vi "Main.vi"(11 "Error in":errorcluster) -> (15 "Error out":errorcluster)   [LabVIEW 2020, in "Automated Teller Machine.lvlib"]
doc: "The ATM will simulate the actual working of a real time ATM machine which stores the customer credentials and the money available in a csv file."
uses:
  Automated Teller Machine.lvlib
  Type_def/Queue_operations.ctl
  Type_def/Queue_Datatype.ctl
  Type_def/Data_Cluster.ctl
  Type_def/Left_menu.ctl
  Type_def/Right_menu.ctl
  Type_def/Left_button.ctl
  Type_def/Right_button.ctl
  <vilib>/Utility/file.llb/Read Delimited Spreadsheet (string).vi
  <vilib>/Utility/file.llb/Write Delimited Spreadsheet (string).vi
panel:
  in  "User input":string
  out "RIGHT MENU":T1
  out "LEFT MENU":T1
  in  "RIGHT BUTTON":T2
  in  "LEFT BUTTON":T3
  out "ATM Message":string
  in  "Enter":bool
  in  "Card Simulator":bool
  # "Automated Teller Machine"
  # "Instrunctions:\n1. Start the machine.\n2. Insert Card.\n3. Enter Account number.\n4. Press Enter.\n5. Enter the operation \nneeded to be performed.\n4. If cash withdrawal or\nadding give the amount\nand press enter."
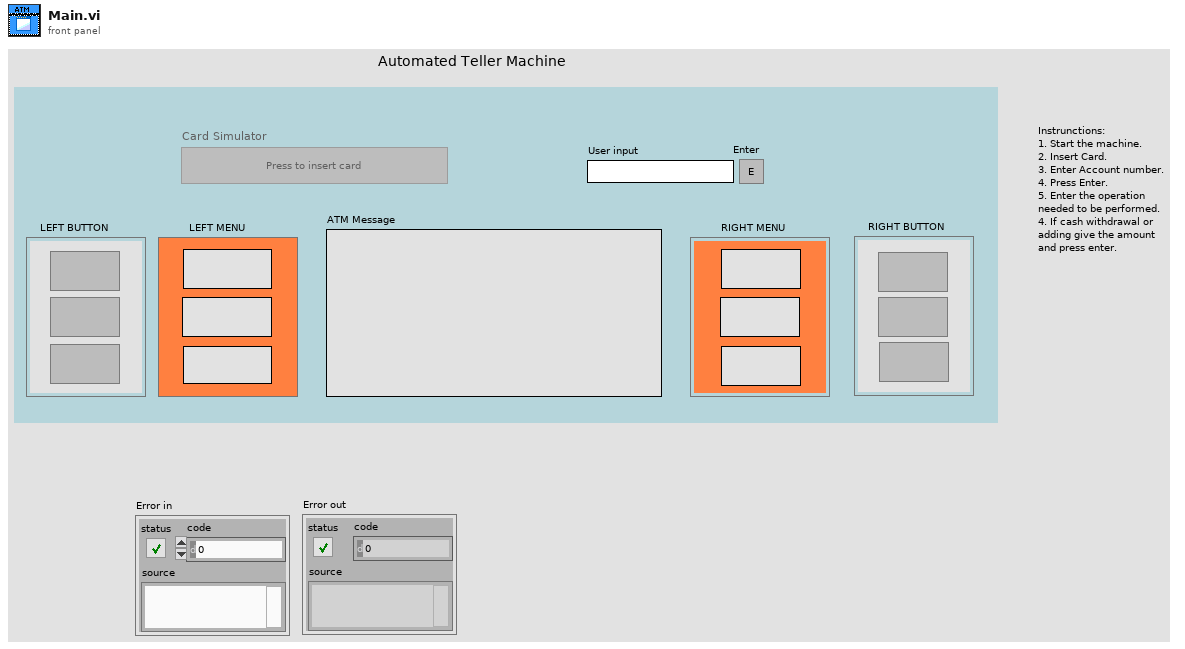
[diagram p1: front panel]
types:
  T1 = cluster{"String":string, "String 2":string, "String 3":string}
  T2 = cluster{"Deposit":bool, "Withdraw":bool, "Fastcash":bool}
  T3 = cluster{"None":bool, "Balance Inquiry":bool, "Returncard":bool}
  T4 = typedef "Automated Teller Machine.lvlib/Data_Cluster.ctl" = cluster{"ATM Message":string, "LEFT MENU":T5, "RIGHT MENU":T6, "LEFT BUTTON":T7, "Enter":bool, "Card Simulator":bool, "RIGHT BUTTON":T8, "start_time":dbl, "file_Path":path, "Account_no_array":string[], "Balance_array":i32[], "_First_Name":string[], "Last_Name":string[], "Card_simulator":enum8{"Enabled", "Disabled", "Disabled and Grayed Out"}, "User_input":enum8{"Enabled", "Disabled", "Disabled and Grayed Out"}, "Enter":enum8{"Enabled", "Disabled", "Disabled and Grayed Out"}, "Left_button":enum8{"Enabled", "Disabled", "Disabled and Grayed Out"}, "Righ_button":enum8{"Enabled", "Disabled", "Disabled and Grayed Out"}, "User_input":string, "Index_postion":i32, "Operation":string, "To_deposit":i32, "To_withdraw":i32, "Start/Stop Timer":bool}
  T5 = typedef "Automated Teller Machine.lvlib/Left_menu.ctl" = cluster{"String":string, "String 2":string, "String 3":string}
  T6 = typedef "Automated Teller Machine.lvlib/Right_menu.ctl" = cluster{"String":string, "String 2":string, "String 3":string}
  T7 = typedef "Automated Teller Machine.lvlib/Left_button.ctl" = cluster{"Boolean":bool, "Boolean 2":bool, "Boolean 3":bool}
  T8 = typedef "Automated Teller Machine.lvlib/Right_button.ctl" = cluster{"Boolean":bool, "Boolean 2":bool, "Boolean 3":bool}
  T9 = typedef "Automated Teller Machine.lvlib/Queue_Datatype.ctl" = cluster{"State":string, "Data":variant}
  T10 = typedef "Automated Teller Machine.lvlib/Queue_operations.ctl" = enum16{"Create", "Enqueue", "Dequeue", "Flush", "Release"}
  T11 = enum8{"Enabled", "Disabled", "Disabled and Grayed Out"}
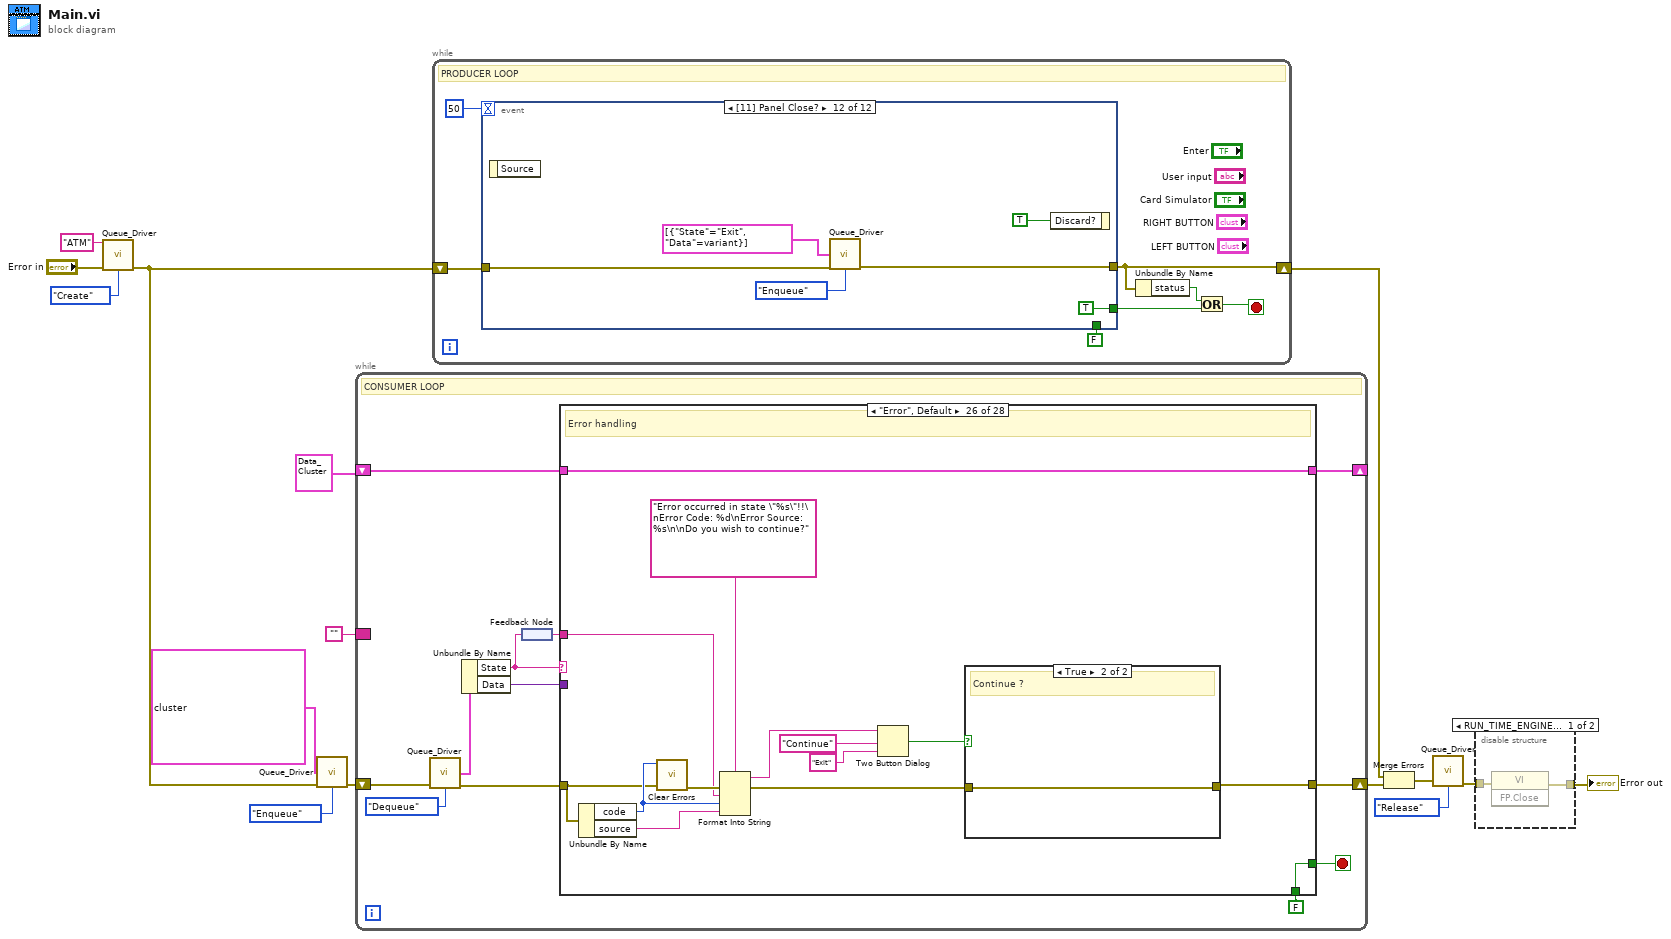
[diagram p0: block diagram]
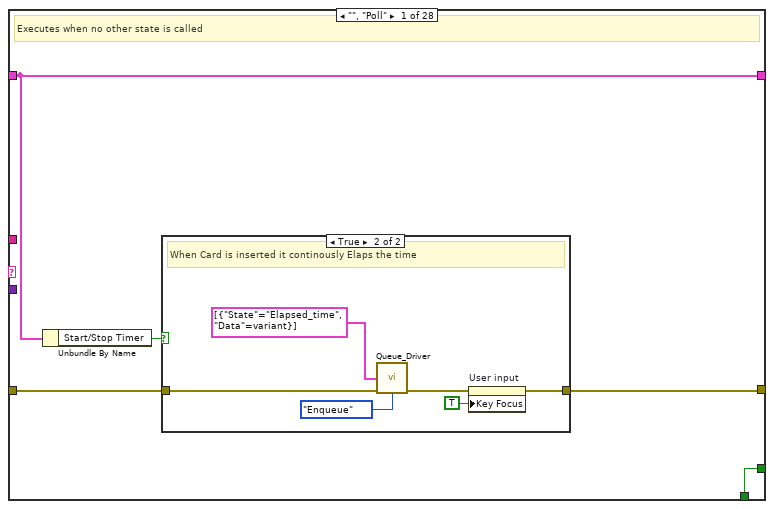
[diagram p3: hidden frame]
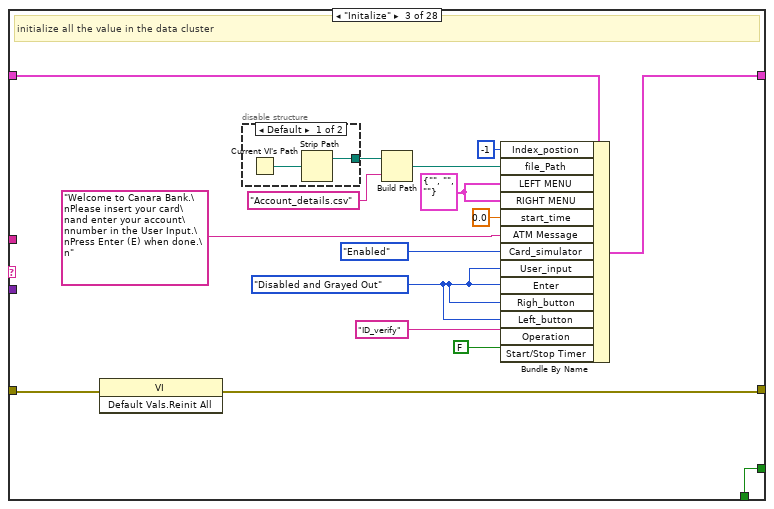
[diagram p6: hidden frame]
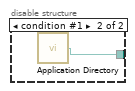
[diagram p7: hidden frame]
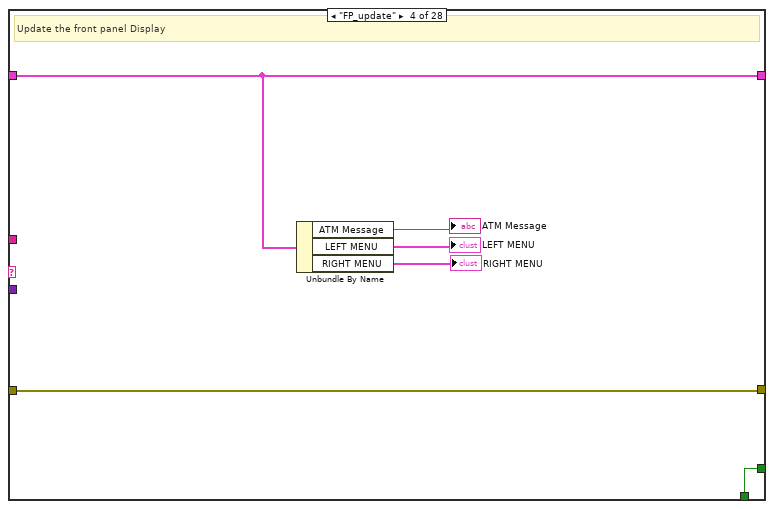
[diagram p8: hidden frame]
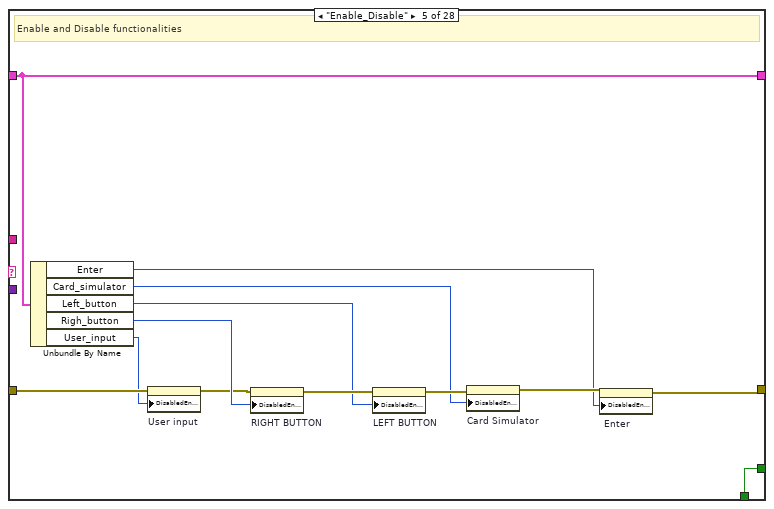
[diagram p9: hidden frame]
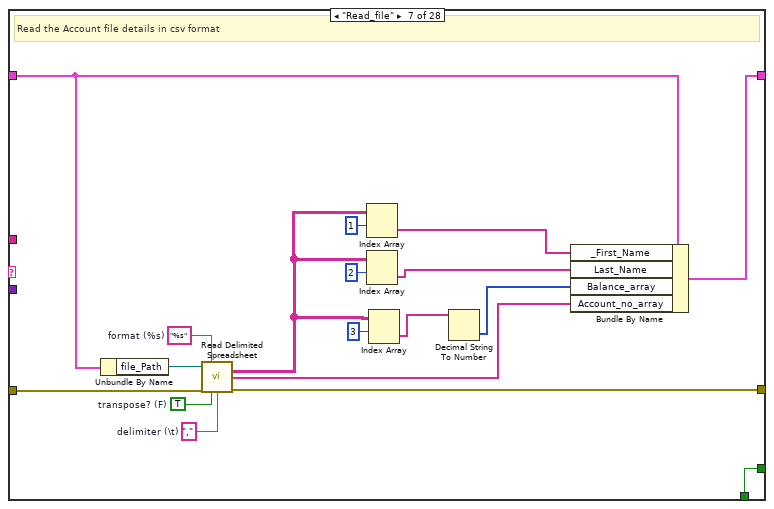
[diagram p11: hidden frame]
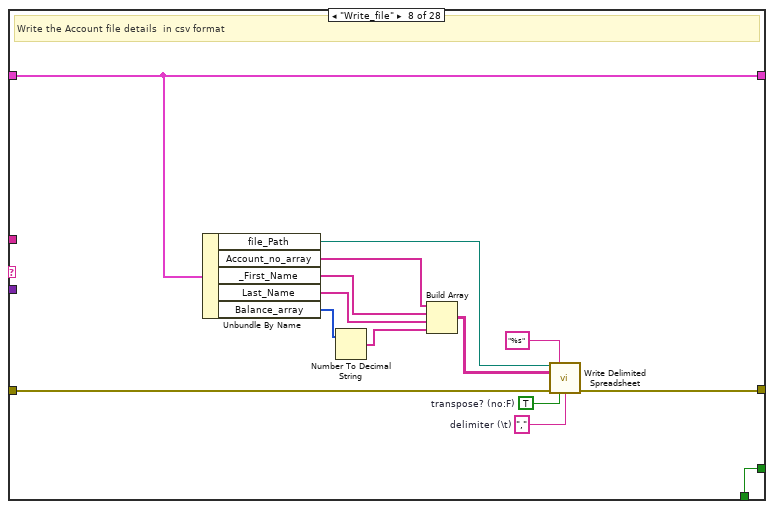
[diagram p12: hidden frame]
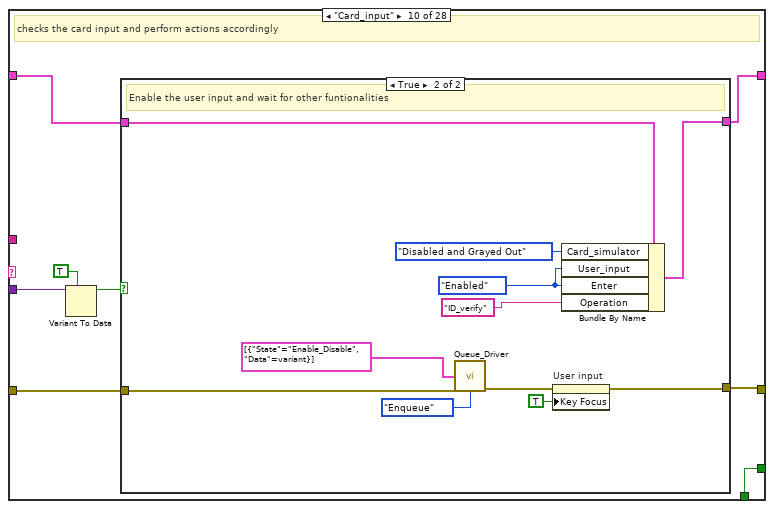
[diagram p14: hidden frame]
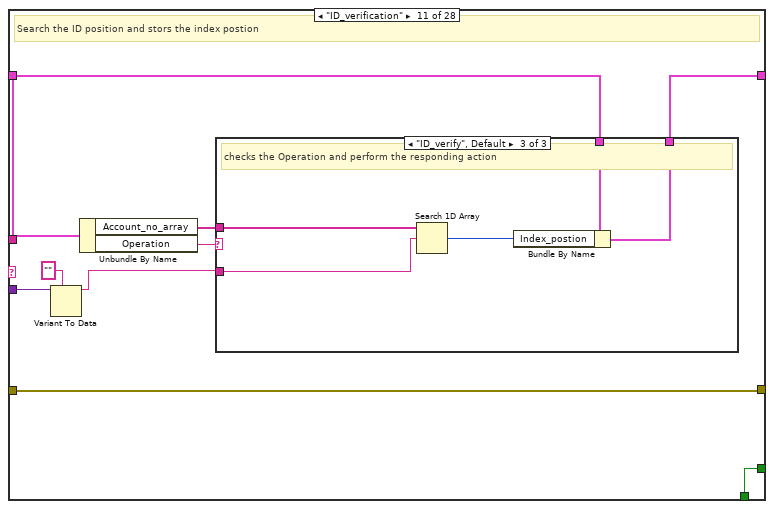
[diagram p16: hidden frame]
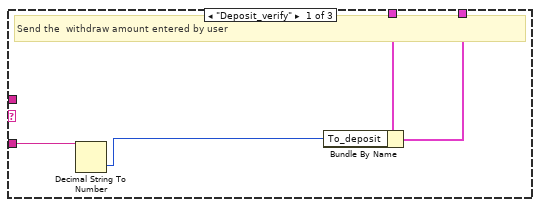
[diagram p17: hidden frame]
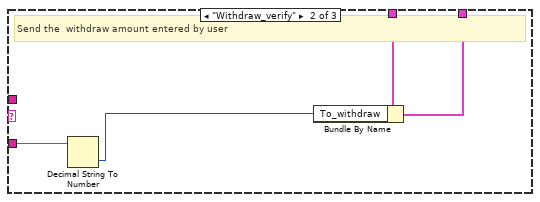
[diagram p18: hidden frame]
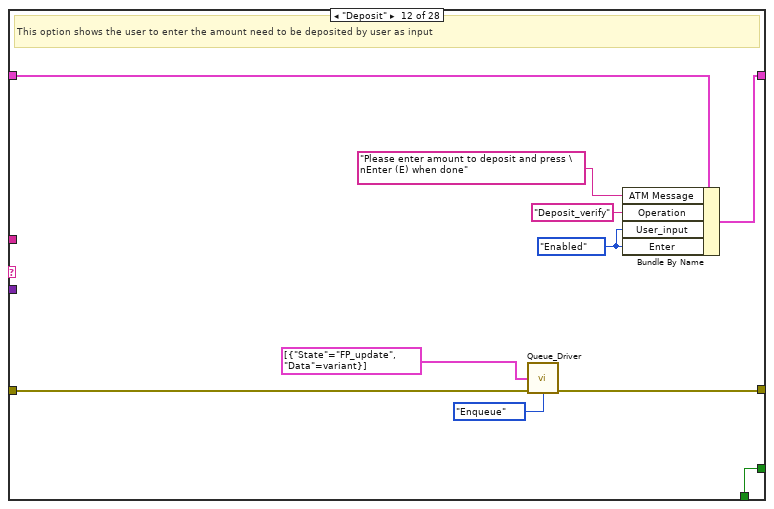
[diagram p19: hidden frame]
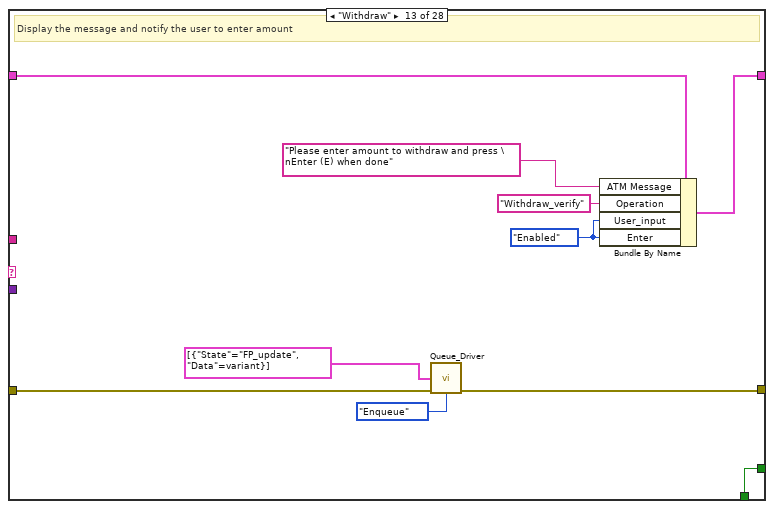
[diagram p20: hidden frame]
diagram:
  n1 = call "Queue_Driver.vi"("Name"="ATM", "Error in"="Error in", "Operation"=Queue_operations."Create") -> ("Error out"=w10:errorcluster)  [unwired: 11 in, 1 out]
  n2 = call "Queue_Driver.vi"("States_Data[]"=T9[] [{"State"="Initalize", "Data"=variant}, {"State"="FP_update", "Data"=variant}, {"State"="Enable_Disable", "Data"=variant}, {"State"="Read_file", "Data"=variant}], "Error in"=w10, "Operation"=Queue_operations."Enqueue") -> ("Error out"=w8:errorcluster)  [unwired: 11 in, 1 out]
  n3 = while {
    shift-right: [w19] -> w6
    shift-left: w8 -> [w23]
    shift-right: [w20] -> _
    shift-left: T4 {"ATM Message"="", "LEFT MENU"={"String"="", "String 2"="", "String 3"=""}, "RIGHT MENU"={"String"="", "String 2"="", "String 3"=""}, "LEFT BUTTON"={"Boolean"=FALSE, "Boolean 2"=FALSE, "Boolean 3"=FALSE}, "Enter"=FALSE, "Card Simulator"=FALSE, "RIGHT BUTTON"={"Boolean"=FALSE, "Boolean 2"=FALSE, "Boolean 3"=FALSE}, "start_time"=0.0, "file_Path"=path "", "Account_no_array"=[], "Balance_array"=[], "_First_Name"=[], "Last_Name"=[], "Card_simulator"=enum."Disabled and Grayed Out", "User_input"=enum."Disabled and Grayed Out", "Enter"=enum."Disabled and Grayed Out", "Left_button"=enum."Disabled and Grayed Out", "Righ_button"=enum."Disabled and Grayed Out", "User_input"="", "Index_postion"=0, "Operation"="", "To_deposit"=0, "To_withdraw"=0, "Start/Stop Timer"=FALSE} -> [w21]
    border: "" -> [_]
    stop <- w26 stop-if-true
    # "CONSUMER LOOP"
    n4 = call "Queue_Driver.vi"("Error in"=w23, "Operation"=Queue_operations."Dequeue") -> ("State_out"=w25:T9, "Error out"=w22:errorcluster)  [unwired: 12 in]
    n5 = Unbundle By Name(w25) -> ("State"=w18:string, "Data"=w24:variant)
    n6 = feedback-in #1(w18) -> ()
    n7 = feedback #1() -> (w17:string)
    n8 = case shown="\"Error\", Default" w18 {
      tunnel: [w28 w40 w43 w62 w68 w81 w84 w102 w116 w119 w140 w162 w172 w182 w192 w195 w212 w244 w259 w290 w303 w311 w314 w321 w336 w339 w358 TRUE] -> w26
      tunnel: w24 -> [_ _ _ _ _ _ _ _ _ w126 w144 _ _ _ _ _ _ _ _ _ _ _ _ _ _ _ _ _]
      tunnel: w22 -> [w32 w41 w48 w63 w72 w82 w99 w115 w117 w121 w141 w167 w176 w185 w193 w198 w216 w250 w267 w293 w305 w312 w320 w326 w337 w343 w359 w364]
      tunnel: [w30 w42 w55 w64 w74 w83 w96 w106 w118 w122 w146 w170 w179 w190 w194 w196 w218 w257 w262 w301 w309 w313 w317 w328 w338 w342 w360 w362] -> w20
      tunnel: w21 -> [w30 w42 w56 w64 w74 w83 w97 w106 w118 w123 w147 w171 w181 w191 w194 w196 w219 w258 w263 w302 w310 w313 w318 w328 w338 w342 w360 w362]
      tunnel: [w31 w41 w49 w63 w73 w82 w86 w105 w117 w120 w141 w168 w175 w184 w193 w197 w215 w249 w266 w292 w304 w312 w320 w325 w337 w341 w359 w361] -> w19
      tunnel: w17 -> [_ _ _ _ _ _ _ _ _ _ _ _ _ _ _ _ _ _ _ _ _ _ _ _ _ w340 _ _]
      tunnel: FALSE -> [w28 w40 w43 w62 w68 w81 w84 w102 w116 w119 w140 w162 w172 w182 w192 w195 w212 w244 w259 w290 w303 w311 w314 w321 w336 w339 w358 _]
      frame "", "Poll" {
        # "Executes when no other state is called"
        n9 = Unbundle By Name(w30) -> ("Start/Stop Timer"=w29:bool)
        n10 = case shown="True" w29 {
          tunnel: w32 -> [w33 w39]
          tunnel: [w33 w34] -> w31
          frame False {
            # "Wait for the time to start"
          }
          frame True {
            # "When Card is inserted it continously Elaps the time"
            n11 = call "Queue_Driver.vi"("States_Data[]"=T9[] [{"State"="Elapsed_time", "Data"=variant}], "Error in"=w39, "Operation"=Queue_operations."Enqueue") -> ("Error out"=w35:errorcluster)  [unwired: 11 in, 1 out]
            n12 = property on="User input" class="Str"(error in=w35, "Key Focus"=TRUE) -> (error out=w34:errorcluster)  [unwired: 1 in, 1 out]
          }
        }
      }
      frame "/***Initalization***/" {
      }
      frame "Initalize" {
        w44 = T5 {"String"="", "String 2"="", "String 3"=""} ("LEFT MENU")
        w45 = T11."Disabled and Grayed Out" ("User_input")
        # "initialize all the value in the data cluster"
        n13 = invoke class="VI" method="Default Vals.Reinit All"(error in=w48) -> (error out=w49:errorcluster)  [unwired: 2 in, 2 out]
        n14 = disable-structure shown="Default" {
          disable-tunnel: [w59 w61] -> w58
          frame condition #0 (active) {
            n15 = Current VI's Path() -> (path=w60:path)
            n16 = Strip Path(path=w60) -> (stripped path=w59:path)  [unwired: 1 out]
          }
          frame condition #1 {
            n17 = call <vilib>:"Application Directory.vi"() -> ("Application Directory"=w61:path)
          }
        }
        n18 = Build Path(base path=w58, name or relative path="Account_details.csv") -> (appended path=w54:path)
        n19 = Bundle By Name(cluster=w56, "Index_postion"=-1, "file_Path"=w54, "LEFT MENU"=w44, "RIGHT MENU"=w44, "start_time"=0.0, "ATM Message"="Welcome to Canara Bank.\nPlease insert your card\nand enter your account\nnumber in the User Input.\nPress Enter (E) when done.\n", "Card_simulator"=T11."Enabled", "User_input"=w45, "Enter"=w45, "Righ_button"=w45, "Left_button"=w45, "Operation"="ID_verify", "Start/Stop Timer"=FALSE) -> (w55:T4)
      }
      frame "FP_update" {
        # "Update the front panel Display"
        n20 = Unbundle By Name(w64) -> ("ATM Message"=→"ATM Message":string, "LEFT MENU"=→"LEFT MENU":T5, "RIGHT MENU"=→"RIGHT MENU":T6)
      }
      frame "Enable_Disable" {
        # "Enable and Disable functionalities"
        n21 = Unbundle By Name(w74) -> ("Enter"=w69:T11, "Card_simulator"=w75:T11, "Left_button"=w76:T11, "Righ_button"=w77:T11, "User_input"=w70:T11)
        n22 = property on="User input" class="Str"(error in=w72, "DisabledEnum"=w70) -> (error out=w71:errorcluster)  [unwired: 1 in, 1 out]
        n23 = property on="RIGHT BUTTON" class="Clust"(error in=w71, "DisabledEnum"=w77) -> (error out=w80:errorcluster)  [unwired: 1 in, 1 out]
        n24 = property on="LEFT BUTTON" class="Clust"(error in=w80, "DisabledEnum"=w76) -> (error out=w79:errorcluster)  [unwired: 1 in, 1 out]
        n25 = property on="Card Simulator" class="Bool (strict)"(error in=w79, "DisabledEnum"=w75) -> (error out=w78:errorcluster)  [unwired: 1 in, 1 out]
        n26 = property on="Enter" class="Bool"(error in=w78, "DisabledEnum"=w69) -> (error out=w73:errorcluster)  [unwired: 1 in, 1 out]
      }
      frame "/***file_handling***/" {
      }
      frame "Read_file" {
        w95 = TRUE  # transpose? (F)
        w98 = "%s"  # format (%s)
        w100 = ","  # delimiter (\t)
        # "Read the Account file details in csv format"
        n27 = Unbundle By Name(w97) -> ("file_Path"=w101:path)
        n28 = call-poly <vilib>:"Read Delimited Spreadsheet.vi"("file path (dialog if empty)"=w101, "format (%s)"=w98, "error in (no error)"=w99, "transpose? (F)"=w95, "delimiter (\\t)"=w100) -> ("all rows"=w90:string[][], "first row"=w85:string[], "error out"=w86:errorcluster)  [unwired: 5 in, 3 out]
        n29 = Index Array(array=w90, index (row)=1) -> (element=w88:string[])  [unwired: 1 in]
        n30 = Index Array(array=w90, index (row)=2) -> (element=w87:string[])  [unwired: 1 in]
        n31 = Index Array(array=w90, index (row)=3) -> (element=w93:string[])  [unwired: 1 in]
        n32 = Decimal String To Number(string=w93) -> (number=w92:i32[])  [unwired: 2 in, 1 out]
        n33 = Bundle By Name(cluster=w97, "_First_Name"=w88, "Last_Name"=w87, "Balance_array"=w92, "Account_no_array"=w85) -> (w96:T4)
      }
      frame "Write_file" {
        w103 = TRUE  # transpose? (no:F)
        w114 = ","  # delimiter (\t)
        # "Write the Account file details  in csv format"
        n34 = Unbundle By Name(w106) -> ("file_Path"=w113:path, "Account_no_array"=w104:string[], "_First_Name"=w112:string[], "Last_Name"=w111:string[], "Balance_array"=w110:i32[])
        n35 = Number To Decimal String(number=w110) -> (decimal integer string=w109:string[])  [unwired: 1 in]
        n36 = Build Array(w104, w112, w111, w109) -> (w108:string[][])
        n37 = call-poly <vilib>:"Write Delimited Spreadsheet.vi"("file path (dialog if empty)"=w113, "format (%s)"="%s", "2D data"=w108, "error in (no error)"=w115, "transpose? (no:F)"=w103, "delimiter (\\t)"=w114) -> ("error out"=w105:errorcluster)  [unwired: 8 in, 1 out]
      }
      frame "/***ATM_Operations***/" {
      }
      frame "Card_input" {
        # "checks the card input and perform actions accordingly"
        n38 = Variant To Data(type=TRUE, Variant=w126) -> (data=w124:bool)  [unwired: 1 in, 1 out]
        n39 = case shown="True" w124 {
          tunnel: w123 -> [w127 w139]
          tunnel: [w127 w138] -> w122
          tunnel: w121 -> [w128 w135]
          tunnel: [w128 w129] -> w120
          frame False {
            # "Locks the ATM card untill the card is released"
          }
          frame True {
            w133 = T11."Enabled" ("User_input")
            # "Enable the user input and wait for other funtionalities"
            n40 = call "Queue_Driver.vi"("States_Data[]"=T9[] [{"State"="Enable_Disable", "Data"=variant}], "Error in"=w135, "Operation"=Queue_operations."Enqueue") -> ("Error out"=w130:errorcluster)  [unwired: 11 in, 1 out]
            n41 = property on="User input" class="Str"(error in=w130, "Key Focus"=TRUE) -> (error out=w129:errorcluster)  [unwired: 1 in, 1 out]
            n42 = Bundle By Name(cluster=w139, "Card_simulator"=T11."Disabled and Grayed Out", "User_input"=w133, "Enter"=w133, "Operation"="ID_verify") -> (w138:T4)
          }
        }
      }
      frame "ID_verification" {
        # "Search the ID position and stors the index postion"
        n43 = Variant To Data(type="", Variant=w144) -> (data=w142:string)  [unwired: 1 in, 1 out]
        n44 = Unbundle By Name(w147) -> ("Account_no_array"=w148:string[], "Operation"=w145:string)
        n45 = case shown="\"ID_verify\", Default" w145 {
          tunnel: w148 -> [_ _ w161]
          tunnel: w147 -> [w152 w155 w160]
          tunnel: [w151 w154 w159] -> w146
          tunnel: w142 -> [w150 w156 w157]
          frame "Deposit_verify" {
            # "Send the  withdraw amount entered by user"
            n46 = Decimal String To Number(string=w150) -> (number=w149:i32)  [unwired: 2 in, 1 out]
            n47 = Bundle By Name(cluster=w152, "To_deposit"=w149) -> (w151:T4)
          }
          frame "Withdraw_verify" {
            # "Send the  withdraw amount entered by user"
            n48 = Decimal String To Number(string=w156) -> (number=w153:i32)  [unwired: 2 in, 1 out]
            n49 = Bundle By Name(cluster=w155, "To_withdraw"=w153) -> (w154:T4)
          }
          frame "ID_verify", Default {
            # "checks the Operation and perform the responding action"
            n50 = Search 1D Array(1D array=w161, element=w157) -> (index of element=w158:i32)  [unwired: 1 in]
            n51 = Bundle By Name(cluster=w160, "Index_postion"=w158) -> (w159:T4)
          }
        }
      }
      frame "Deposit" {
        w163 = T11."Enabled" ("Enter")
        # "This option shows the user to enter the amount need to be deposited by user as input"
        n52 = call "Queue_Driver.vi"("States_Data[]"=T9[] [{"State"="FP_update", "Data"=variant}], "Error in"=w167, "Operation"=Queue_operations."Enqueue") -> ("Error out"=w168:errorcluster)  [unwired: 11 in, 1 out]
        n53 = Bundle By Name(cluster=w171, "ATM Message"="Please enter amount to deposit and press \nEnter (E) when done", "Operation"="Deposit_verify", "User_input"=w163, "Enter"=w163) -> (w170:T4)
      }
      frame "Withdraw" {
        w173 = T11."Enabled" ("Enter")
        # "Display the message and notify the user to enter amount"
        n54 = call "Queue_Driver.vi"("States_Data[]"=T9[] [{"State"="FP_update", "Data"=variant}], "Error in"=w176, "Operation"=Queue_operations."Enqueue") -> ("Error out"=w175:errorcluster)  [unwired: 11 in, 1 out]
        n55 = Bundle By Name(cluster=w181, "ATM Message"="Please enter amount to withdraw and press \nEnter (E) when done", "Operation"="Withdraw_verify", "User_input"=w173, "Enter"=w173) -> (w179:T4)
      }
      frame "Withdraw_50" {
        w183 = T11."Disabled and Grayed Out" ("User_input")
        # "Fast cash automatically withdraw 50 Dollar cash to user if exisits"
        n56 = call "Queue_Driver.vi"("States_Data[]"=T9[] [{"State"="Enter_function", "Data"=variant}], "Error in"=w185, "Operation"=Queue_operations."Enqueue") -> ("Error out"=w184:errorcluster)  [unwired: 11 in, 1 out]
        n57 = Bundle By Name(cluster=w191, "To_withdraw"=50, "Operation"="Withdraw_verify", "User_input"=w183, "Enter"=w183) -> (w190:T4)
      }
      frame "/***Enter_operations***/" {
      }
      frame "Enter_function" {
        # "Based on the operation happened the enter function moves to state"
        n58 = Unbundle By Name(w196) -> ("Operation"=w199:string)
        n59 = case shown="\"Withdraw_verify\"" w199 {
          tunnel: w198 -> [w201 w207 w211]
          tunnel: [w200 w206 w210] -> w197
          frame "Withdraw_verify" {
            n60 = call "Queue_Driver.vi"("States_Data[]"=T9[] [{"State"="Check_withdraw", "Data"=variant}], "Error in"=w201, "Operation"=Queue_operations."Enqueue") -> ("Error out"=w200:errorcluster)  [unwired: 11 in, 1 out]
          }
          frame "Deposit_verify" {
            n61 = call "Queue_Driver.vi"("States_Data[]"=T9[] [{"State"="Check_deposit", "Data"=variant}], "Error in"=w207, "Operation"=Queue_operations."Enqueue") -> ("Error out"=w206:errorcluster)  [unwired: 11 in, 1 out]
          }
          frame "ID_verify", Default {
            n62 = call "Queue_Driver.vi"("States_Data[]"=T9[] [{"State"="Check_ID", "Data"=variant}], "Error in"=w211, "Operation"=Queue_operations."Enqueue") -> ("Error out"=w210:errorcluster)  [unwired: 11 in, 1 out]
          }
        }
      }
      frame "Check_ID" {
        # "Display the information if the account exisits"
        n63 = Unbundle By Name(w219) -> ("_First_Name"=w217:string[], "Index_postion"=w213:i32, "Last_Name"=w214:string[])
        n64 = Greater Or Equal To 0?(x=w213) -> (x >= 0?=w220:bool)
        n65 = case shown="True" w220 {
          tunnel: w219 -> [w227 w242]
          tunnel: [w226 w241] -> w218
          tunnel: w217 -> [_ w239]
          tunnel: w213 -> [_ w235]
          tunnel: [w224 w233] -> w215
          tunnel: w216 -> [w223 w232]
          tunnel: w214 -> [_ w234]
          frame False {
            n66 = call "Queue_Driver.vi"("States_Data[]"=T9[] [{"State"="FP_update", "Data"=variant}], "Error in"=w223, "Operation"=Queue_operations."Enqueue") -> ("Error out"=w224:errorcluster)  [unwired: 11 in, 1 out]
            n67 = Bundle By Name(cluster=w227, "ATM Message"="Account Information Incorrect\nPlease Re-Enter Account Number.\nPress Enter (E) when done\n") -> (w226:T4)
          }
          frame True {
            w228 = T11."Enabled" ("Left_button")
            n68 = Index Array(array=w239, index=w235) -> (element=w238:string)
            n69 = Index Array(array=w234, index=w235) -> (element=w237:string)
            n70 = call "Queue_Driver.vi"("States_Data[]"=T9[] [{"State"="FP_update", "Data"=variant}, {"State"="Enable_Disable", "Data"=variant}], "Error in"=w232, "Operation"=Queue_operations."Enqueue") -> ("Error out"=w233:errorcluster)  [unwired: 11 in, 1 out]
            n71 = Format Into String(format string="Welcome to ICICI Bank\n%s %s\nPlease select transaction\nby using the buttons", w238, w237) -> (resulting string=w240:string)  [unwired: 2 in, 1 out]
            n72 = Bundle By Name(cluster=w242, "ATM Message"=w240, "LEFT MENU"=T1 {"String"="None", "String 2"="Balance Inquiry", "String 3"="Return Card and Terminate"}, "RIGHT MENU"=T1 {"String"="Deposit", "String 2"="Withdraw", "String 3"="Fast cash  -  $50"}, "Righ_button"=w228, "Left_button"=w228) -> (w241:T4)
          }
        }
      }
      frame "Check_deposit" {
        # "After the Deposit is done the acount balance is updated"
        n73 = Unbundle By Name(w258) -> ("Balance_array"=w256:i32[], "Index_postion"=w254:i32, "To_deposit"=w245:i32)
        n74 = Index Array(array=w256, index=w254) -> (element=w246:i32)
        n75 = Add(x=w246, y=w245) -> (x+y=w251:i32)
        n76 = call "Queue_Driver.vi"("States_Data[]"=T9[] [{"State"="Write_file", "Data"=variant}, {"State"="FP_update", "Data"=variant}], "Error in"=w250, "Operation"=Queue_operations."Enqueue") -> ("Error out"=w249:errorcluster)  [unwired: 11 in, 1 out]
        n77 = Format Into String(format string="$%d is Deposited", w245) -> (resulting string=w253:string)  [unwired: 2 in, 1 out]
        n78 = Replace Array Subset(array=w256, new element=w251, index=w254) -> (w255:i32[])
        n79 = Bundle By Name(cluster=w258, "ATM Message"=w253, "Balance_array"=w255) -> (w257:T4)
      }
      frame "Check_withdraw" {
        # "the Entered amount is checked for withdraw process"
        n80 = Unbundle By Name(w263) -> ("Balance_array"=w261:i32[], "Index_postion"=w260:i32, "To_withdraw"=w264:i32)
        n81 = Index Array(array=w261, index=w260) -> (element=w265:i32)
        n82 = Greater Or Equal?(x=w265, y=w264) -> (x >= y?=w268:bool)
        n83 = case shown="False" w268 {
          tunnel: w267 -> [w270 w287]
          tunnel: [w269 w286] -> w266
          tunnel: w265 -> [_ w285]
          tunnel: w264 -> [_ w277]
          tunnel: w263 -> [w275 w284]
          tunnel: [w274 w283] -> w262
          tunnel: w261 -> [_ w282]
          tunnel: w260 -> [_ w281]
          frame False {
            # "Notify the user about the insufficient balance"
            n84 = call "Queue_Driver.vi"("States_Data[]"=T9[] [{"State"="FP_update", "Data"=variant}], "Error in"=w270, "Operation"=Queue_operations."Enqueue") -> ("Error out"=w269:errorcluster)  [unwired: 11 in, 1 out]
            n85 = Bundle By Name(cluster=w275, "ATM Message"="Insufficient funds in account\nPlease check your balance\nand try again") -> (w274:T4)
          }
          frame True {
            # "Withdraw if the amount exisits"
            n86 = Subtract(x=w285, y=w277) -> (x-y=w280:i32)
            n87 = Replace Array Subset(array=w282, new element=w280, index=w281) -> (w279:i32[])
            n88 = Format Into String(format string="$ %d  Withdrawn" ("ATM Message"), w277) -> (resulting string=w276:string)  [unwired: 2 in, 1 out]
            n89 = Bundle By Name(cluster=w284, "ATM Message"=w276, "Balance_array"=w279) -> (w283:T4)
            n90 = call "Queue_Driver.vi"("States_Data[]"=T9[] [{"State"="Write_file", "Data"=variant}, {"State"="FP_update", "Data"=variant}], "Error in"=w287, "Operation"=Queue_operations."Enqueue") -> ("Error out"=w286:errorcluster)  [unwired: 11 in, 1 out]
          }
        }
      }
      frame "Check_balance" {
        w291 = T11."Disabled and Grayed Out" ("User_input")
        # "Displays the message of the bank balance on the account number"
        n91 = Unbundle By Name(w302) -> ("Balance_array"=w300:i32[], "Index_postion"=w299:i32)
        n92 = Index Array(array=w300, index=w299) -> (element=w297:i32)
        n93 = Format Into String(format string="Your Balance Is:\n$ %d", w297) -> (resulting string=w296:string)  [unwired: 2 in, 1 out]
        n94 = call "Queue_Driver.vi"("States_Data[]"=T9[] [{"State"="FP_update", "Data"=variant}, {"State"="Enable_Disable", "Data"=variant}], "Error in"=w293, "Operation"=Queue_operations."Enqueue") -> ("Error out"=w292:errorcluster)  [unwired: 11 in, 1 out]
        n95 = Bundle By Name(cluster=w302, "ATM Message"=w296, "User_input"=w291, "Enter"=w291) -> (w301:T4)
      }
      frame "Return_card" {
        # "This option terminate the program and button will turn off"
        n96 = call "Queue_Driver.vi"("States_Data[]"=T9[] [{"State"="FP_update", "Data"=variant}, {"State"="Exit", "Data"=variant}], "Error in"=w305, "Operation"=Queue_operations."Enqueue") -> ("Error out"=w304:errorcluster)  [unwired: 11 in, 1 out]
        n97 = Bundle By Name(cluster=w310, "ATM Message"="Your session has been terminated\ndue to inactivity or menu selection.\nPlease take your card\nGoodbye") -> (w309:T4)
      }
      frame "/***Timer_function***/" {
      }
      frame "Start_time" {
        n98 = Get Date/Time In Seconds() -> (seconds since 1Jan1904=w319:timestamp)
        n99 = To Double Precision Float(number=w319) -> (double precision float=w316:dbl)
        n100 = Bundle By Name(cluster=w318, "start_time"=w316, "Start/Stop Timer"=TRUE) -> (w317:T4)
      }
      frame "Elapsed_time" {
        n101 = Unbundle By Name(w328) -> ("start_time"=w327:dbl)
        n102 = Get Date/Time In Seconds() -> (seconds since 1Jan1904=w330:timestamp)
        n103 = To Double Precision Float(number=w330) -> (double precision float=w329:dbl)
        n104 = Subtract(x=w329, y=w327) -> (x-y=w322:dbl)
        n105 = Greater?(x=w322, y=10.0 ("x")) -> (0:w324:bool)
        n106 = case shown="True" w324 {
          tunnel: w326 -> [w331 w335]
          tunnel: [w331 w334] -> w325
          frame False {
          }
          frame True {
            n107 = call "Queue_Driver.vi"("States_Data[]"=T9[] [{"State"="Initalize", "Data"=variant}, {"State"="FP_update", "Data"=variant}, {"State"="Enable_Disable", "Data"=variant}, {"State"="Read_file", "Data"=variant}], "Error in"=w335, "Operation"=Queue_operations."Enqueue") -> ("Error out"=w334:errorcluster)  [unwired: 11 in, 1 out]
          }
        }
      }
      frame "/***Error_handling***/" {
      }
      frame "Error", Default {
        # "Error handling"
        n108 = Unbundle By Name(w343) -> ("code"=w350:i32, "source"=w349:string)
        n109 = call <vilib>:"Clear Errors.vi"("error in (no error)"=w343, "specific error code to clear (0: all)"=w350) -> ("error out"=w352:errorcluster)  [unwired: 4 in, 1 out]
        n110 = Format Into String(format string="Error occurred in state \"%s\"!!\nError Code: %d\nError Source: %s\n\nDo you wish to continue?", error in=w352, w340, w350, w349) -> (resulting string=w348:string, error out=w344:errorcluster)  [unwired: 1 in]
        n111 = Two Button Dialog(message=w348, 1:"Exit" ("F button name (\"Cancel\")"), 2:"Continue" ("T button name (\"OK\")")) -> (T button?=w345:bool)
        n112 = case shown="True" w345 {
          tunnel: w344 -> [w356 w357]
          tunnel: [w355 w357] -> w341
          frame False {
            # "Exit to stop the Simulation"
            n113 = call "Queue_Driver.vi"("States_Data[]"=T9[] [{"State"="Exit", "Data"=variant}], "Error in"=w356, "Operation"=Queue_operations."Enqueue") -> ("Error out"=w355:errorcluster)  [unwired: 11 in, 1 out]
          }
          frame True {
            # "Continue ?"
          }
        }
      }
      frame "/***Exit***/" {
      }
      frame "Exit" {
        # "Exit the program"
        n114 = call "Queue_Driver.vi"("Error in"=w364, "Operation"=Queue_operations."Flush") -> ("Error out"=w361:errorcluster)  [unwired: 12 in, 1 out]
      }
    }
  }
  n115 = while {
    shift-right: [w370] -> w7
    shift-left: w10 -> [w372]
    stop <- w367 stop-if-true
    # "PRODUCER LOOP"
    n116 = event shown="[11] Panel Close?" {
      selector: _ -> [_ _ _ _ _ _ _ _ _ _ _ _]
      dyn-events: _ -> [_ _ _ _ _ _ _ _ _ _ _ _]
      timeout: 50 -> [_ _ _ _ _ _ _ _ _ _ _ _]
      tunnel: [w373 w375 w387 w399 w412 w418 w423 TRUE w435 w440 w445 TRUE] -> w368
      tunnel: w372 -> [w374 w376 w398 w403 w413 w422 w425 w429 w436 w441 w447 w451]
      tunnel: [w374 w386 w397 w401 w417 w421 w424 w432 w439 w442 w446 w450] -> w370
      tunnel: FALSE -> [w373 w375 w387 w399 w412 w418 w423 _ w435 w440 w445 _]
      event Timeout {
        n117 = event-data() -> ()  [unwired: 1 in, 1 out]
      }
      event "Card Simulator": Value Change {
        w379 = T9 {"State"="", "Data"=variant}
        n118 = event-data() -> ("NewVal"=w381:bool)  [unwired: 1 in]
        n119 = To Variant(anything=w381) -> (Variant=w380:variant)
        n120 = Bundle By Name(cluster=w379, "State"="Card_input", "Data"=w380) -> (w384:T9)
        n121 = Bundle By Name(cluster=w379, "State"="Start_time") -> (w378:T9)
        n122 = Build Array(w378, w384) -> (w383:T9[])
        n123 = call "Queue_Driver.vi"("States_Data[]"=w383, "Error in"=w376, "Operation"=Queue_operations."Enqueue") -> ("Error out"=w386:errorcluster)  [unwired: 11 in, 1 out]
      }
      event "User input": Value Change {
        w389 = T9 {"State"="", "Data"=variant}
        n124 = event-data() -> ("NewVal"=w394:string)  [unwired: 1 in]
        n125 = To Variant(anything=w394) -> (Variant=w393:variant)
        n126 = Bundle By Name(cluster=w389, "State"="ID_verification", "Data"=w393) -> (w392:T9)
        n127 = Bundle By Name(cluster=w389, "State"="Start_time") -> (w388:T9)
        n128 = Build Array(w388, w392) -> (w391:T9[])
        n129 = call "Queue_Driver.vi"("States_Data[]"=w391, "Error in"=w398, "Operation"=Queue_operations."Enqueue") -> ("Error out"=w397:errorcluster)  [unwired: 11 in, 1 out]
      }
      event "User input": Key Down? {
        # "This Event to filter the User input When the user try\nto type Alphabets in keyboard"
        n130 = event-data() -> ("Char"=w409:i16)  [unwired: 1 in]
        n131 = Equal?(x=w409, y=i16 8) -> (x = y?=w406:bool)
        n132 = In Range and Coerce(upper limit=i16 58, x=w409, lower limit=i16 48) -> (In Range?=w407:bool)  [unwired: 1 out]
        n133 = Or(x=w407, y=w406) -> (x .or. y?=w405:bool)
        n134 = Not(x=w405) -> (.not. x?=w404:bool)
        n135 = call "Queue_Driver.vi"("States_Data[]"=T9[] [{"State"="Start_time", "Data"=variant}], "Error in"=w403, "Operation"=Queue_operations."Enqueue") -> ("Error out"=w401:errorcluster)  [unwired: 11 in, 1 out]
        n136 = event-data("Discard?"=w404) -> ()  [unwired: 1 in, 1 out]
      }
      event "Enter": Value Change {
        n137 = event-data() -> ()  [unwired: 1 in, 1 out]
        n138 = invoke on="User input" class="Str" method="Reinit To Default"(error in=w413) -> (error out=w414:errorcluster)  [unwired: 2 in, 2 out]
        n139 = call "Queue_Driver.vi"("States_Data[]"=T9[] [{"State"="Enter_function", "Data"=variant}, {"State"="Start_time", "Data"=variant}], "Error in"=w414, "Operation"=Queue_operations."Enqueue") -> ("Error out"=w417:errorcluster)  [unwired: 11 in, 1 out]
      }
      event "LEFT BUTTON.Balance Inquiry": Value Change {
        n140 = event-data() -> ()  [unwired: 1 in, 1 out]
        n141 = call "Queue_Driver.vi"("States_Data[]"=T9[] [{"State"="Check_balance", "Data"=variant}, {"State"="Start_time", "Data"=variant}], "Error in"=w422, "Operation"=Queue_operations."Enqueue") -> ("Error out"=w421:errorcluster)  [unwired: 11 in, 1 out]
      }
      event "LEFT BUTTON.None": Value Change {
        n142 = event-data() -> ()  [unwired: 1 in, 1 out]
        n143 = call "Queue_Driver.vi"("States_Data[]"=T9[] [{"State"="Start_time", "Data"=variant}], "Error in"=w425, "Operation"=Queue_operations."Enqueue") -> ("Error out"=w424:errorcluster)  [unwired: 11 in, 1 out]
      }
      event "LEFT BUTTON.Returncard": Value Change {
        n144 = event-data() -> ()  [unwired: 1 in, 1 out]
        n145 = property on="Card Simulator" class="Bool (strict)"(error in=w429, "Value"=FALSE ("Card Simulator")) -> (error out=w430:errorcluster)  [unwired: 1 in, 1 out]
        n146 = call "Queue_Driver.vi"("States_Data[]"=T9[] [{"State"="Return_card", "Data"=variant}], "Error in"=w430, "Operation"=Queue_operations."Enqueue") -> ("Error out"=w432:errorcluster)  [unwired: 11 in, 1 out]
      }
      event "RIGHT BUTTON.Deposit": Value Change {
        n147 = event-data() -> ()  [unwired: 1 in, 1 out]
        n148 = call "Queue_Driver.vi"("States_Data[]"=T9[] [{"State"="Deposit", "Data"=variant}, {"State"="Start_time", "Data"=variant}], "Error in"=w436, "Operation"=Queue_operations."Enqueue") -> ("Error out"=w439:errorcluster)  [unwired: 11 in, 1 out]
      }
      event "RIGHT BUTTON.Withdraw": Value Change {
        n149 = event-data() -> ()  [unwired: 1 in, 1 out]
        n150 = call "Queue_Driver.vi"("States_Data[]"=T9[] [{"State"="Withdraw", "Data"=variant}, {"State"="Start_time", "Data"=variant}], "Error in"=w441, "Operation"=Queue_operations."Enqueue") -> ("Error out"=w442:errorcluster)  [unwired: 11 in, 1 out]
      }
      event "RIGHT BUTTON.Fastcash": Value Change {
        n151 = event-data() -> ()  [unwired: 1 in, 1 out]
        n152 = call "Queue_Driver.vi"("States_Data[]"=T9[] [{"State"="Withdraw_50", "Data"=variant}, {"State"="Start_time", "Data"=variant}], "Error in"=w447, "Operation"=Queue_operations."Enqueue") -> ("Error out"=w446:errorcluster)  [unwired: 11 in, 1 out]
      }
      event Panel Close? {
        n153 = event-data() -> ()  [unwired: 1 in, 1 out]
        n154 = call "Queue_Driver.vi"("States_Data[]"=T9[] [{"State"="Exit", "Data"=variant}], "Error in"=w451, "Operation"=Queue_operations."Enqueue") -> ("Error out"=w450:errorcluster)  [unwired: 11 in, 1 out]
        n155 = event-data("Discard?"=TRUE) -> ()  [unwired: 1 in, 1 out]
      }
    }
    n156 = Unbundle By Name(w370) -> ("status"=w369:bool)
    n157 = Or(x=w369, y=w368) -> (x .or. y?=w367:bool)
  }
  n158 = Merge Errors(w7, w6) -> (w5:errorcluster)
  n159 = call "Queue_Driver.vi"("Error in"=w5, "Operation"=Queue_operations."Release") -> ("Error out"=w3:errorcluster)  [unwired: 12 in, 1 out]
  n160 = disable-structure shown="RUN_TIME_ENGINE==True" {
    disable-tunnel: w3 -> [w457 w458]
    disable-tunnel: [w456 w458] -> w2
    frame condition #0 {
      n161 = invoke class="VI" method="FP.Close"(error in=w457) -> (error out=w456:errorcluster)  [unwired: 2 in, 2 out]
    }
    frame condition #1 (active) {
    }
  }
  "Error out" <- w2
